vi "SALINAS_DAVID_ESPINOZA_CESAR.vi"() -> ()   [LabVIEW 2025]
uses:
  <vilib>/express/express arith-compare/Formula/XNode/ExpressFormulaBlockNode.xnode
panel:
  out "CALIENTE":bool
  out "FRIO":bool
  in  "stop":bool
  out "KELVIN":dbl
  out "FAHRENHEIT":dbl
  out "CELSIUS":dbl
  out "KELVIN":dbl(knob) scale=273.0..373.0
  out "FAHRENHEIT":dbl(knob) scale=32.0..212.0
  out "CELSIUS":dbl(knob) scale=0.0..100.0
  in  "Slide":dbl(slide) scale=0.0..100.0
  out "KELVIN":dbl(slide) scale=273.0..373.0
  out "FAHRENHEIT":dbl(slide) scale=32.0..212.0
  out "CELSIUS":dbl(slide) scale=0.0..100.0
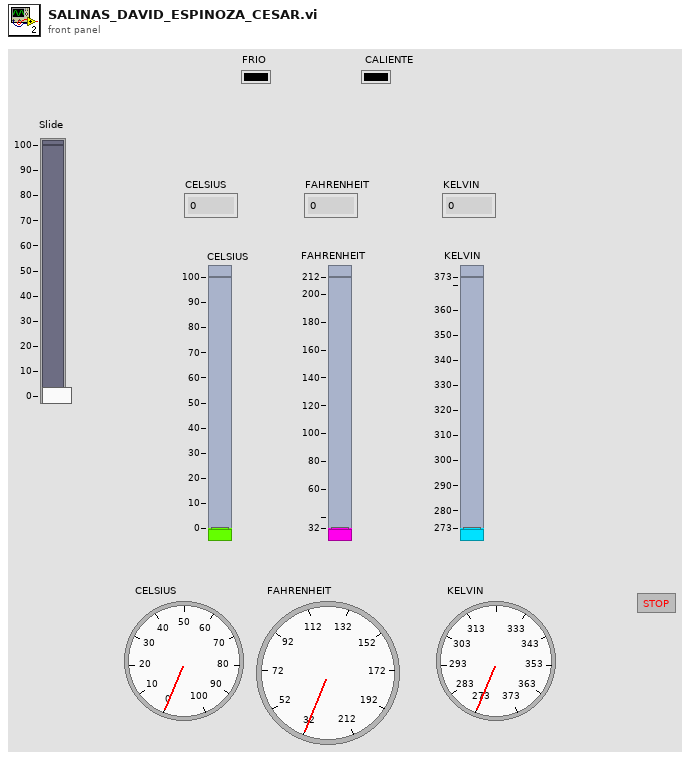
[diagram p1: front panel]
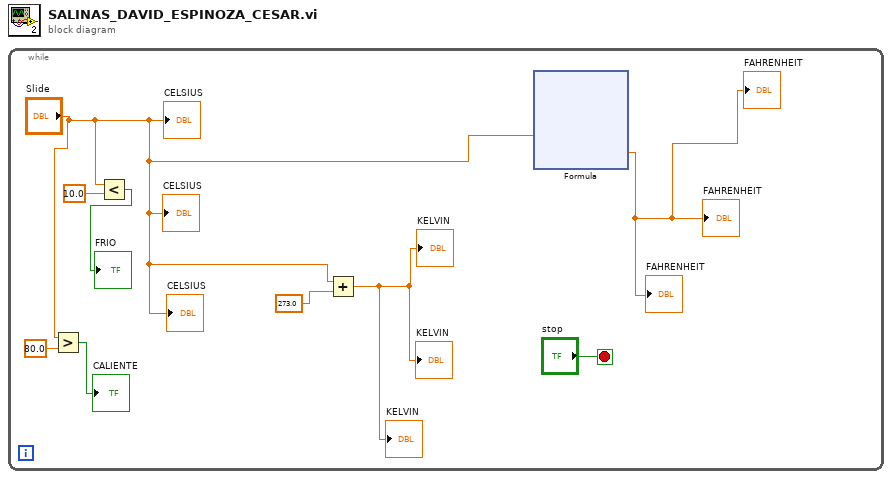
[diagram p0: block diagram]
diagram:
  n1 = while {
    stop <- "stop" stop-if-true
    n2 = Greater?(x="Slide", y=80.0) -> (0:→"CALIENTE":bool)
    n3 = Less?(x="Slide", y=10.0) -> (x < y?=→"FRIO":bool)
    n4 = Add(x="Slide", y=273.0) -> (x+y=→"KELVIN" →"KELVIN" →"KELVIN":dbl)
    n5 = xnode "Formula"("X1"="Slide") -> ("Result"=→"FAHRENHEIT" →"FAHRENHEIT" →"FAHRENHEIT":dbl)  [unwired: 1 in, 1 out]
    "CELSIUS" <- "Slide"
    "CELSIUS" <- "Slide"
    "CELSIUS" <- "Slide"
  }
